vi "Compile - Rx Buffered Channel Refs.vi"(6 "Packet Name":string, 8 "error in (no error)":errorcluster, 11 "Item Ref in":T1 format="%.0x") -> (0 "error out":errorcluster, 3 "Item Ref out":T1 format="%.0x", 4 "Rx Ref Array":T2(array[cluster]) {"VS Refs" format="%.0x"})   [LabVIEW 2019, in "UDP-Custom-Device System Explorer.lvlib"]
uses:
  UDP-Custom-Device System Explorer.lvlib
  <vilib>/NI VeriStand/Custom Device API/Custom Device Item Ref.ctl
  <vilib>/NI VeriStand/Custom Device API/Custom Device API.lvlib
  Property Accessors/Buffered Data Packet.lvlib
  <vilib>/NI VeriStand/Custom Device Tools/Custom Device Utility Library/Custom Device Utility Library.lvlib
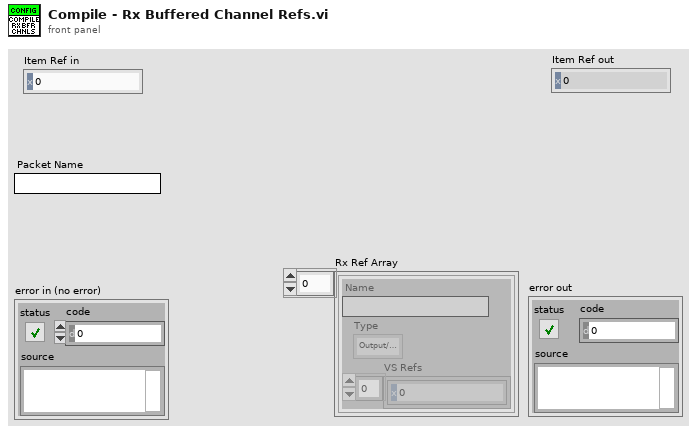
[diagram p1: front panel]
types:
  T1 = typedef "Custom Device API.lvlib/Custom Device Item Ref.ctl" = u64
  T2 = cluster{"Name":string, "Type":enum16{"Output/Write", "Input/Read", "Input/ReadWrite"}, "VS Refs":T1[]}[]
  T3 = cluster{"Name":string, "Type":enum16{"Output/Write", "Input/Read", "Input/ReadWrite"}, "VS Refs":T1[]}
  T4 = enum16{"Output/Write", "Input/Read", "Input/ReadWrite"}
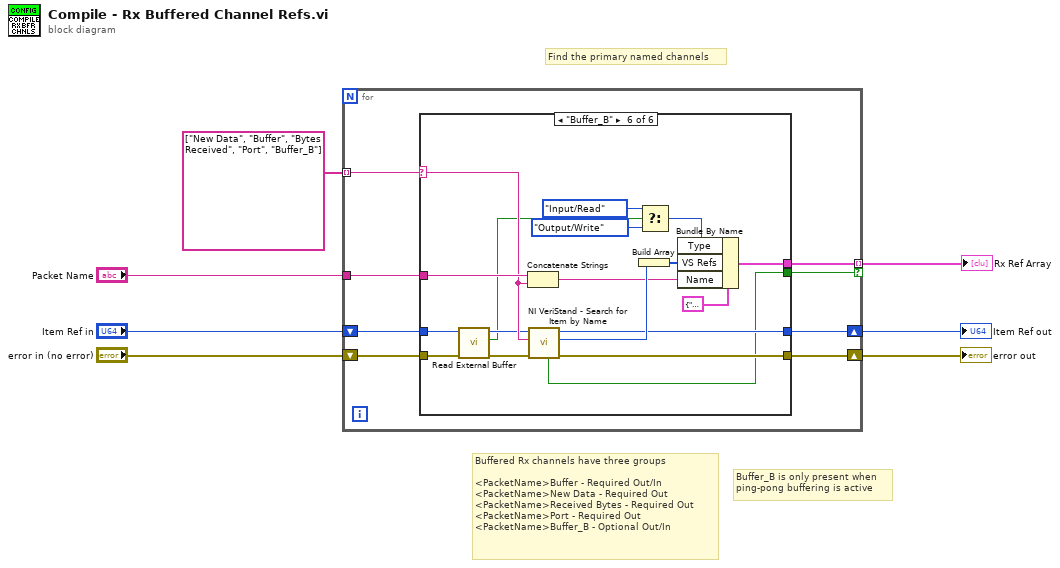
[diagram p0: block diagram]
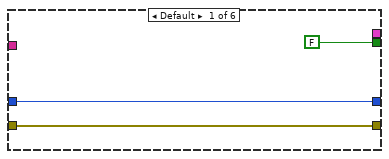
[diagram p2: hidden frame]
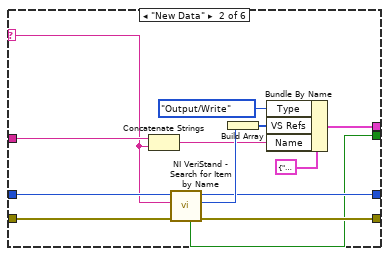
[diagram p3: hidden frame]
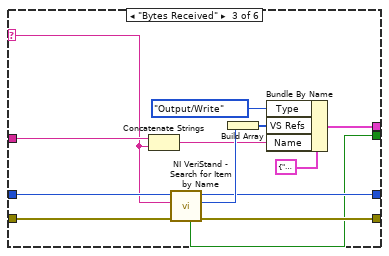
[diagram p4: hidden frame]
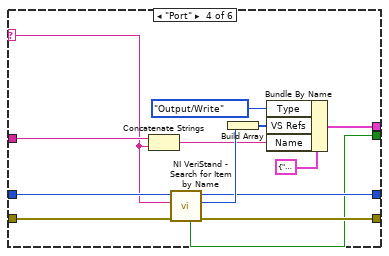
[diagram p5: hidden frame]
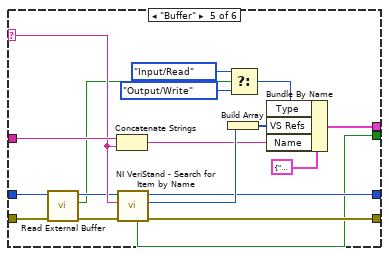
[diagram p6: hidden frame]
diagram:
  # "Buffer_B is only present when\nping-pong buffering is active"
  # "Find the primary named channels"
  # "Buffered Rx channels have three groups\n\n<PacketName>Buffer - Required Out/In\n<PacketName>New Data - Required Out\n<PacketName>Received Bytes - Required Out\n<PacketName>Port - Required Out\n<PacketName>Buffer_B - Optional Out/In"
  n1 = for {
    tunnel: string[] ["New Data", "Buffer", "Bytes Received", "Port", "Buffer_B"] ("Item GUID") -> [w15] mode=indexing
    tunnel: "Packet Name" -> [w10]
    tunnel: [w12] -> w4 mode=indexing if=w11
    shift-right: [w9] -> w6
    shift-left: "Item Ref in" -> [w13]
    shift-right: [w8] -> w5
    shift-left: "error in (no error)" -> [w14]
    n2 = case shown="\"Buffer_B\"" w15 {
      selector: w15 -> [_ w20 w33 w46 w67 w85]
      tunnel: w14 -> [w17 w26 w39 w52 w65 w83]
      tunnel: w13 -> [w18 w27 w40 w53 w63 w81]
      tunnel: [w18 w25 w38 w51 w72 w90] -> w9
      tunnel: [w17 w24 w37 w50 w71 w89] -> w8
      tunnel: [_ w23 w36 w49 w70 w88] -> w12
      tunnel: [FALSE ("Found") w22 w35 w48 w69 w87] -> w11
      tunnel: w10 -> [_ w21 w34 w47 w68 w86]
      frame Default {
      }
      frame "New Data" {
        n3 = Concatenate Strings(w21, w20) -> (w19:string)
        n4 = call <vilib>:"NI VeriStand - Search for Item by Name.vi"("error in"=w26, "Item Name"=w20, "Section Ref in"=w27) -> ("error out"=w24:errorcluster, "Item Ref"=w29:T1, "Section Ref out"=w25:T1, "Found"=w22:bool)  [unwired: 5 in]
        n5 = Build Array(w29) -> (w30:T1[])
        n6 = Bundle By Name(cluster=T3 {"Name"="", "Type"=enum."Output/Write", "VS Refs"=[]} ("Group"), "Type"=T4."Output/Write", "VS Refs"=w30, "Name"=w19) -> (w23:T3)
      }
      frame "Bytes Received" {
        n7 = Concatenate Strings(w34, w33) -> (w32:string)
        n8 = call <vilib>:"NI VeriStand - Search for Item by Name.vi"("error in"=w39, "Item Name"=w33, "Section Ref in"=w40) -> ("error out"=w37:errorcluster, "Item Ref"=w42:T1, "Section Ref out"=w38:T1, "Found"=w35:bool)  [unwired: 5 in]
        n9 = Build Array(w42) -> (w43:T1[])
        n10 = Bundle By Name(cluster=T3 {"Name"="", "Type"=enum."Output/Write", "VS Refs"=[]} ("Group"), "Type"=T4."Output/Write", "VS Refs"=w43, "Name"=w32) -> (w36:T3)
      }
      frame "Port" {
        n11 = Concatenate Strings(w47, w46) -> (w45:string)
        n12 = call <vilib>:"NI VeriStand - Search for Item by Name.vi"("error in"=w52, "Item Name"=w46, "Section Ref in"=w53) -> ("error out"=w50:errorcluster, "Item Ref"=w55:T1, "Section Ref out"=w51:T1, "Found"=w48:bool)  [unwired: 5 in]
        n13 = Build Array(w55) -> (w56:T1[])
        n14 = Bundle By Name(cluster=T3 {"Name"="", "Type"=enum."Output/Write", "VS Refs"=[]} ("Group"), "Type"=T4."Output/Write", "VS Refs"=w56, "Name"=w45) -> (w49:T3)
      }
      frame "Buffer" {
        n15 = call "Read External Buffer.vi"("error in (no error)"=w65, "Node Ptr"=w63) -> ("error out"=w64:errorcluster, "External Buffer"=w59:bool, "Node Ptr out"=w62:T1)  [unwired: 7 in]
        n16 = Concatenate Strings(w68, w67) -> (w66:string)
        n17 = call <vilib>:"NI VeriStand - Search for Item by Name.vi"("error in"=w64, "Item Name"=w67, "Section Ref in"=w62) -> ("error out"=w71:errorcluster, "Item Ref"=w74:T1, "Section Ref out"=w72:T1, "Found"=w69:bool)  [unwired: 5 in]
        n18 = Build Array(w74) -> (w75:T1[])
        n19 = Select(t=T4."Input/Read" ("Type"), s=w59, f=T4."Output/Write" ("Type")) -> (s? t:f=w58:T4)
        n20 = Bundle By Name(cluster=T3 {"Name"="", "Type"=enum."Output/Write", "VS Refs"=[]} ("Group"), "Type"=w58, "VS Refs"=w75, "Name"=w66) -> (w70:T3)
      }
      frame "Buffer_B" {
        n21 = call "Read External Buffer.vi"("error in (no error)"=w83, "Node Ptr"=w81) -> ("error out"=w82:errorcluster, "External Buffer"=w77:bool, "Node Ptr out"=w80:T1)  [unwired: 7 in]
        n22 = Concatenate Strings(w86, w85) -> (w84:string)
        n23 = call <vilib>:"NI VeriStand - Search for Item by Name.vi"("error in"=w82, "Item Name"=w85, "Section Ref in"=w80) -> ("error out"=w89:errorcluster, "Item Ref"=w92:T1, "Section Ref out"=w90:T1, "Found"=w87:bool)  [unwired: 5 in]
        n24 = Build Array(w92) -> (w93:T1[])
        n25 = Select(t=T4."Input/Read" ("Type"), s=w77, f=T4."Output/Write" ("Type")) -> (s? t:f=w76:T4)
        n26 = Bundle By Name(cluster=T3 {"Name"="", "Type"=enum."Output/Write", "VS Refs"=[]} ("Group"), "Type"=w76, "VS Refs"=w93, "Name"=w84) -> (w88:T3)
      }
    }
  }
  "Rx Ref Array" <- w4
  "error out" <- w5
  "Item Ref out" <- w6
